vi "pos_encoder2displayunit.vi"(8 "error in (no error)":errorcluster, 10 "encoder (unit)":dbl, 11 "Motor in":refnum<class "Motor.lvclass">) -> (0 "error out":errorcluster, 2 "pos in display unit":dbl, 3 "Motor out":refnum<class "Motor.lvclass">)   [LabVIEW 2016, in "Hardware.lvlib" / "Motor.lvlib" / "Motor.lvclass"]
uses:
  <userlib>/Common Components/Hardware/Motor/Motor/Motor.lvclass
  <userlib>/Common Components/Hardware/Motor/Motor/Motor.lvclass/Motor.ctl
  <userlib>/Common Components/Hardware/Motor/Motor/Accessor/Read encoder type.vi
  <userlib>/Common Components/Hardware/Motor/Motor/Accessor/Read unit mode.vi
  <userlib>/Common Components/Hardware/Motor/Motor/Accessor/Read motor pulses per revolution.vi
  <userlib>/Common Components/Hardware/Motor/Motor/Accessor/Read display units per motor rev.vi
  <userlib>/Common Components/Hardware/Motor/Motor/Accessor/Read encoder units ratio.vi
panel:
  # "Note:\nif display unit is \"motor pulse\",\nit really means the pulse unit of the motor,\nNOT the unit of built-in encoder (e.g. in UIRobot)."
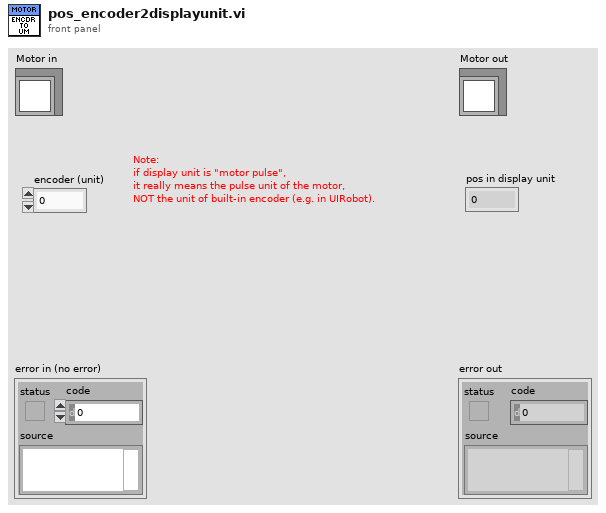
[diagram p1: front panel]
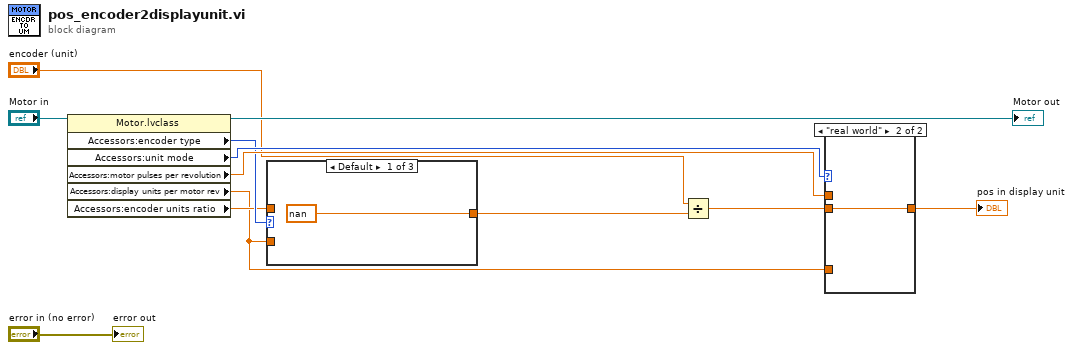
[diagram p0: block diagram]
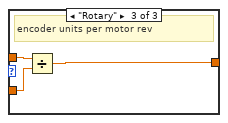
[diagram p3: hidden frame]
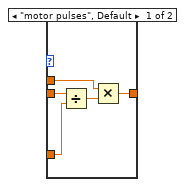
[diagram p4: hidden frame]
diagram:
  n1 = property class="Motor.lvclass"(reference="Motor in") -> (reference out=→"Motor out":refnum<class "Motor.lvclass">, "Accessors:encoder type"=w4:enum16{"Linear", "Rotary"}, "Accessors:unit mode"=w9:enum16{"motor pulses", "real world"}, "Accessors:motor pulses per revolution"=w7:dbl, "Accessors:display units per motor rev"=w1:dbl, "Accessors:encoder units ratio"=w3:dbl)  [unwired: 1 in, 1 out]
  n2 = case shown="Default" w4 {
    tunnel: w3 -> [_ w14 w17]
    tunnel: [nan ("Accessors:encoder units ratio") w14 w15] -> w2
    tunnel: w1 -> [_ _ w16]
    frame Default {
    }
    frame "Linear" {
      # "encoder units per display units"
    }
    frame "Rotary" {
      # "encoder units per motor rev"
      n3 = Divide(x=w17, y=w16) -> (x/y=w15:dbl)
    }
  }
  n4 = Divide(x="encoder (unit)", y=w2) -> (x/y=w6:dbl)
  n5 = case shown="\"real world\"" w9 {
    tunnel: [w20 w23] -> w8
    tunnel: w7 -> [w21 _]
    tunnel: w6 -> [w19 w23]
    tunnel: w1 -> [w18 _]
    frame "motor pulses", Default {
      n6 = Divide(x=w19, y=w18) -> (x/y=w22:dbl)
      n7 = Multiply(x=w21, y=w22) -> (x*y=w20:dbl)
    }
    frame "real world" {
    }
  }
  "pos in display unit" <- w8
  "error out" <- "error in (no error)"
